vi "EJEM13.vi"() -> ()   [LabVIEW 2013]
panel:
  out "Table Control":string[][](table)
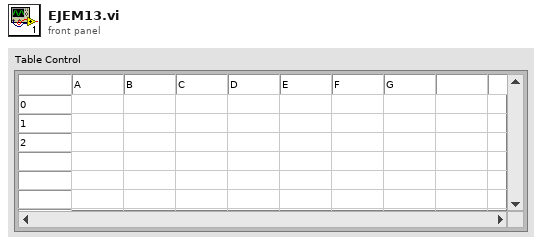
[diagram p1: front panel]
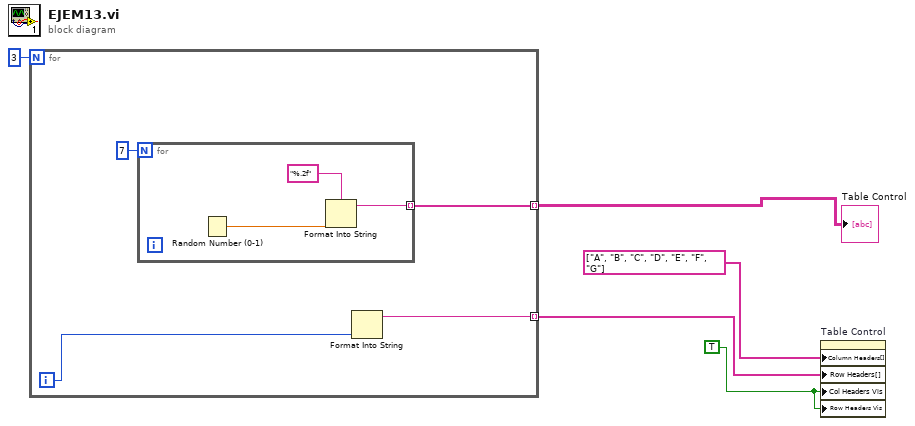
[diagram p0: block diagram]
diagram:
  w3 = TRUE
  n1 = for {
    N: 3 -> [_]
    tunnel: [w7] -> w4 mode=indexing
    tunnel: [w6] -> w1 mode=indexing
    i -> [w8]
    n2 = for {
      N: 7 -> [_]
      tunnel: [w10] -> w7 mode=indexing
      n3 = Random Number (0-1)() -> (number: 0 to 1=w12:dbl)
      n4 = Format Into String(format string="%.2f", w12) -> (resulting string=w10:string)  [unwired: 2 in, 1 out]
    }
    n5 = Format Into String(w8) -> (resulting string=w6:string)  [unwired: 3 in, 1 out]
  }
  "Table Control" <- w4
  n6 = property on="Table Control" class="Tbl (strict)"("Column Headers[]"=string[] ["A", "B", "C", "D", "E", "F", "G"] ("Column Header Strings[]"), "Row Headers[]"=w1, "Col Headers Vis"=w3, "Row Headers Vis"=w3) -> ()  [unwired: 2 in, 2 out]
